vi "RxImgSlice.vi"(8 "error in":errorcluster, 11 "Conn":refnum<k16>) -> (0 "error out":errorcluster, 3 "Data":string)   [LabVIEW 2020]
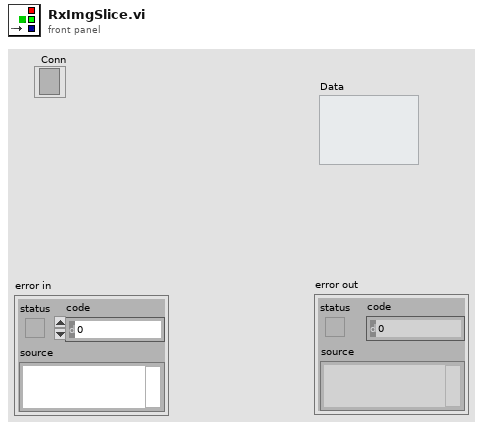
[diagram p1: front panel]
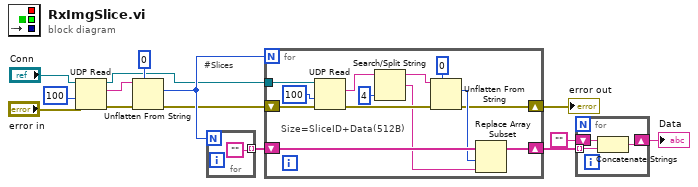
[diagram p0: block diagram]
diagram:
  # "#Slices"
  n1 = UDP Read(connection ID="Conn", timeout ms (25000)=100, 8:"error in") -> (data out=w9:string, error out=w10:errorcluster, 3:w6:refnum<k16>)  [unwired: 3 out]
  n2 = Unflatten From String(type=0, binary string=w9, error in (no error)=w10) -> (value=w8:i32, error out=w5:errorcluster)  [unwired: 3 out]
  n3 = for {
    N: w8 -> [_]
    tunnel: [""] -> w7 mode=indexing
  }
  n4 = for {
    N: w8 -> [_]
    shift-right: [w17] -> w2
    shift-left: w7 -> [w20]
    tunnel: w6 -> [w27]
    shift-right: [w16] -> w3
    shift-left: w5 -> [w26]
    # "Size=SliceID+Data(512B)"
    n5 = UDP Read(connection ID=w27, timeout ms (25000)=100, 8:w26) -> (data out=w22:string, error out=w21:errorcluster)  [unwired: 4 out]
    n6 = Search/Split String(string=w22, offset (0)=4) -> (substring before match=w24:string, match + rest of string=w18:string)  [unwired: 2 out]
    n7 = Unflatten From String(type=0, binary string=w24, error in (no error)=w21) -> (value=w19:i32, error out=w16:errorcluster)  [unwired: 3 out]
    n8 = Replace Array Subset(array=w20, new element=w18, index=w19) -> (w17:string[])
  }
  "error out" <- w3
  n9 = for {
    tunnel: w2 -> [w31] mode=indexing
    shift-right: [w29] -> w1
    shift-left: "" -> [w30]
    n10 = Concatenate Strings(w30, w31) -> (w29:string)
  }
  "Data" <- w1
